vi "Write Element of Serial Commands.vi"(8 "error in (no error)":errorcluster, 9 "String":string, 10 "index":i32, 11 "Arduino in":refnum<class "Arduino.lvclass">) -> (0 "error out":errorcluster, 3 "Arduino out":refnum<class "Arduino.lvclass">)   [LabVIEW 2013, in "Arduino.lvclass"]
uses:
  Arduino.lvclass
  Arduino.lvclass/Arduino.ctl
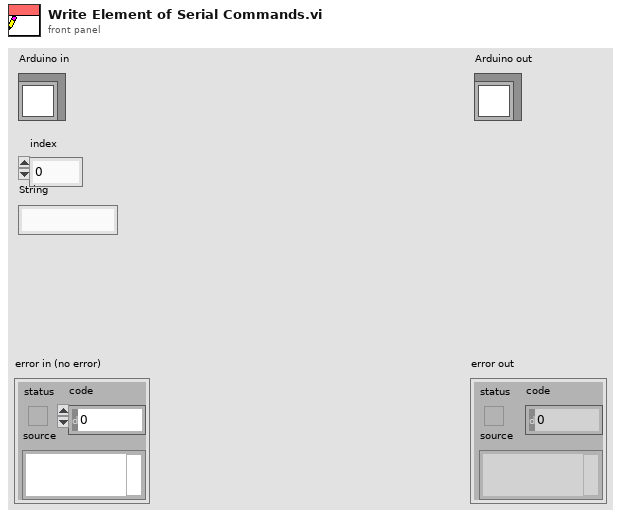
[diagram p1: front panel]
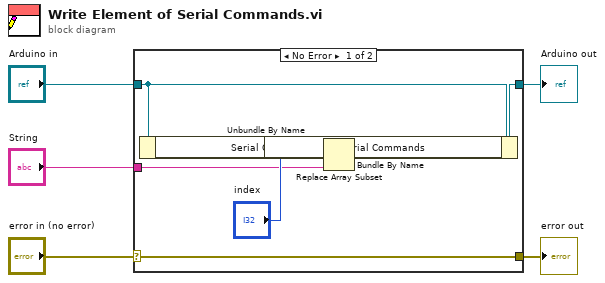
[diagram p0: block diagram]
diagram:
  n1 = case shown="No Error" "error in (no error)" {
    selector: "error in (no error)" -> [w12 w13]
    tunnel: [w12 w13] -> w4
    tunnel: [w11 w14] -> w2
    tunnel: "Arduino in" -> [w10 w14]
    tunnel: "String" -> [w6 _]
    frame No Error {
      n2 = Unbundle By Name(w10) -> ("Serial Commands"=w9:string[])
      n3 = Replace Array Subset(array=w9, new element=w6, index="index") -> (w8:string[])
      n4 = Bundle By Name(cluster=w10, "Serial Commands"=w8) -> (w11:refnum<class "Arduino.lvclass">)
    }
    frame Error {
    }
  }
  "error out" <- w4
  "Arduino out" <- w2
